vi "snr.vi"(8 "error in (no error)":errorcluster, 10 "snr config":T2, 11 "waveform":waveform(dbl)) -> (0 "error out":errorcluster, 3 "SNR data":T1)   [LabVIEW 2019]
uses:
  <vilib>/Waveform/WDTOps.llb/WDT Get Waveform Subset DBL.vi
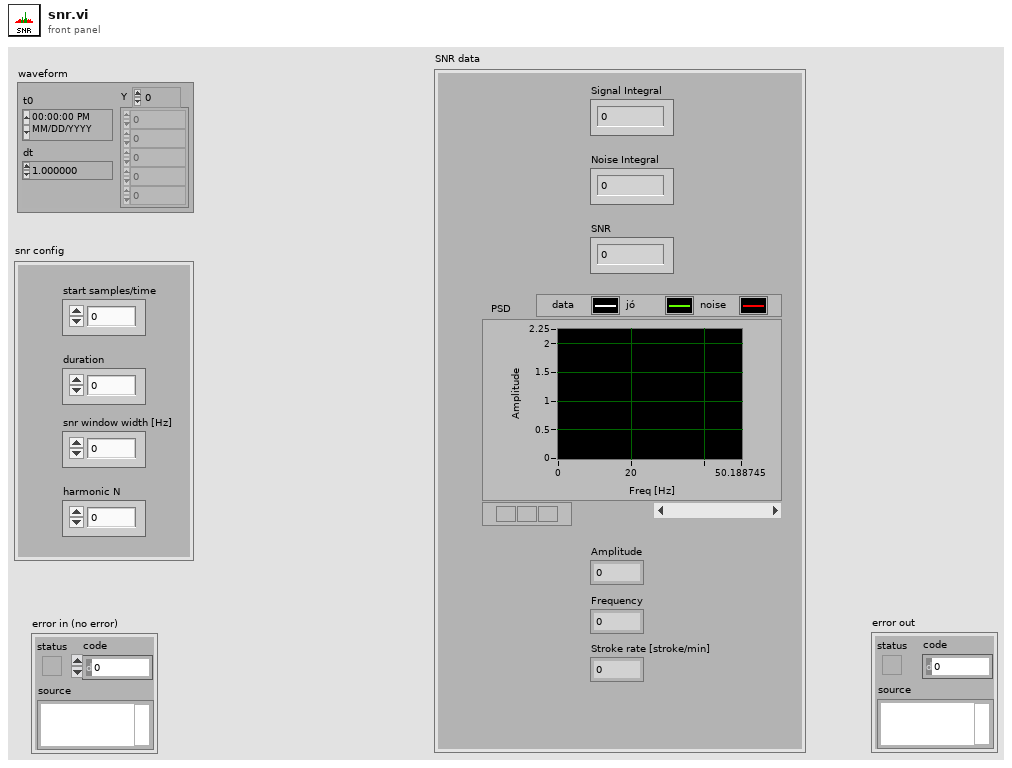
[diagram p1: front panel]
types:
  T1 = cluster{"Signal Integral":dbl, "Noise Integral":dbl, "SNR":dbl, "PSD":cluster{"f0":dbl, "df":dbl, "magnitude":dbl[]}[], "Amplitude":dbl, "Frequency":dbl, "Stroke rate [stroke/min]":dbl}
  T2 = cluster{"start samples/time":dbl, "duration":dbl, "snr window width [Hz]":dbl, "harmonic N":i32}
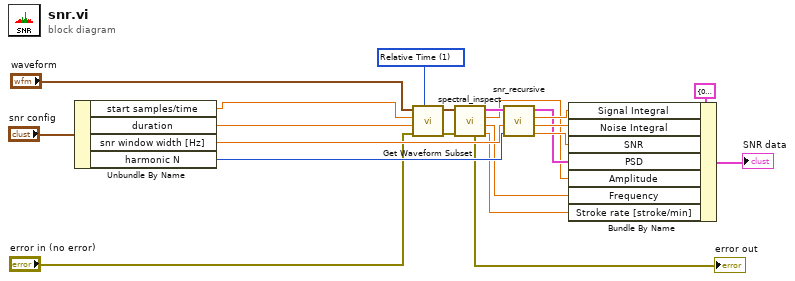
[diagram p0: block diagram]
diagram:
  w18 = u16 1 items=["Samples", "Relative Time"] ("start/duration format")
  n1 = Unbundle By Name("snr config") -> ("start samples/time"=w16:dbl, "duration"=w15:dbl, "snr window width [Hz]"=w13:dbl, "harmonic N"=w14:i32)
  n2 = call-poly <vilib>:"Get Waveform Subset.vi"("start/duration format"=w18, "error in (no error)"="error in (no error)", "duration"=w15, "start samples/time"=w16, "waveform in"="waveform") -> ("error out"=w8:errorcluster, "waveform out"=w19:waveform(dbl))  [unwired: 1 in, 2 out]
  n3 = call "spectral_inspect.vi"("error in (no error)"=w8, "waveform"=w19) -> ("Csapásszám [stroke/min]"=w1:dbl, "freq"=w2:dbl, "amplitude"=w3:dbl, "PSD"=w20:cluster{"f0":dbl, "df":dbl, "magnitude":dbl[]}, "error out"=→"error out":errorcluster)  [unwired: 5 in]
  n4 = call "snr_recursive.vi"("felharmonikus N"=w14, "width [Hz]"=w13, "PSD"=w20) -> ("SNR"=w10:dbl, "Noise Integral"=w11:dbl, "Signal Integral"=w12:dbl, "PSD"=w4:cluster{"f0":dbl, "df":dbl, "magnitude":dbl[]}[])  [unwired: 5 in]
  n5 = Bundle By Name(cluster=T1 {"Signal Integral"=0.0, "Noise Integral"=0.0, "SNR"=0.0, "PSD"=[], "Amplitude"=0.0, "Frequency"=0.0, "Stroke rate [stroke/min]"=0.0} ("SNR data 2"), "Signal Integral"=w12, "Noise Integral"=w11, "SNR"=w10, "PSD"=w4, "Amplitude"=w3, "Frequency"=w2, "Stroke rate [stroke/min]"=w1) -> (→"SNR data":T1)
